vi "TimeTag_LSW_edits_June16.vi"() -> ()   [LabVIEW 2015]
doc: "This sample project is built upon the standard state machine template and shows how you could create an application that acquires, analyzes, and presents data. It includes functionality for presenting configuration dialogs, preserving settings between executions, loading and saving data, as well as exporting graph images and text files.\n\nIt is most appropriate for data that is acquired instantly as it does not allow for screen updates mid acquisition nor does it allow for continuous streaming to disk."
uses:
  <vilib>/ptbypt/NI_PtbyPt.lvlib
panel:
  in  "Averaging":dbl
  in  "Runs":dbl=100.0
  in  "Pulse TTL 2":bool
  in  "Pulse TTL 1":bool
  in  "Toggle\nTTL 2":bool
  in  "Toggle\nTTL 1":bool
  out "Total Starts":dbl
  in  "Record data":bool
  out "Initial time":dbl
  out "Elapsed time (s)":dbl
  out "FPGA_Run Status":dbl
  out "USB_Open Status":dbl
  out "Channel 4 Total\nCounts":dbl
  out "Channel 3 Total\nCounts":dbl
  out "Channel 2 Total\nCounts":dbl
  out "Channel 1 Total\nCounts":dbl
  in  "File Name":string="C:\\FPGA\\test.txt"
  out "?":dbl
  out "?":dbl
  out "?":dbl
  out "?":dbl
  out "stats":i64[](array[numeric])
  in  "Stop":bool
  out "Channel 4 CPS":dbl(knob) scale=0.0..600.0
  out "Channel 3 CPS":dbl(knob) scale=0.0..600.0
  out "Channel 2 CPS":dbl(knob) scale=0.0..600.0
  out "Channel 1 CPS":dbl(knob) scale=0.0..600.0
  # "Starts"
  # "Channel 1"
  # "Channel 2"
  # "Channel 3"
  # "Channel 4"
  # "Coincidence Channels 1 & 2"
  # "Coincidence Channels 1 & 3"
  # "Coincidence Channels 1 & 4"
  # "Coincidence Channels 2 & 3"
  # "Coincidence Channels 2 & 4"
  # "Coincidence Channels 3 & 4"
  # "Coincidence Channels 1 & 2 & 3"
  # "Coincidence Channels 1 & 2 & 4"
  # "Coincidence Channels 1 & 3 & 4"
  # "Coincidence Channels 2 & 3 & 4"
  # "Coincidence Channels 1 & 2 & 3 & 4"
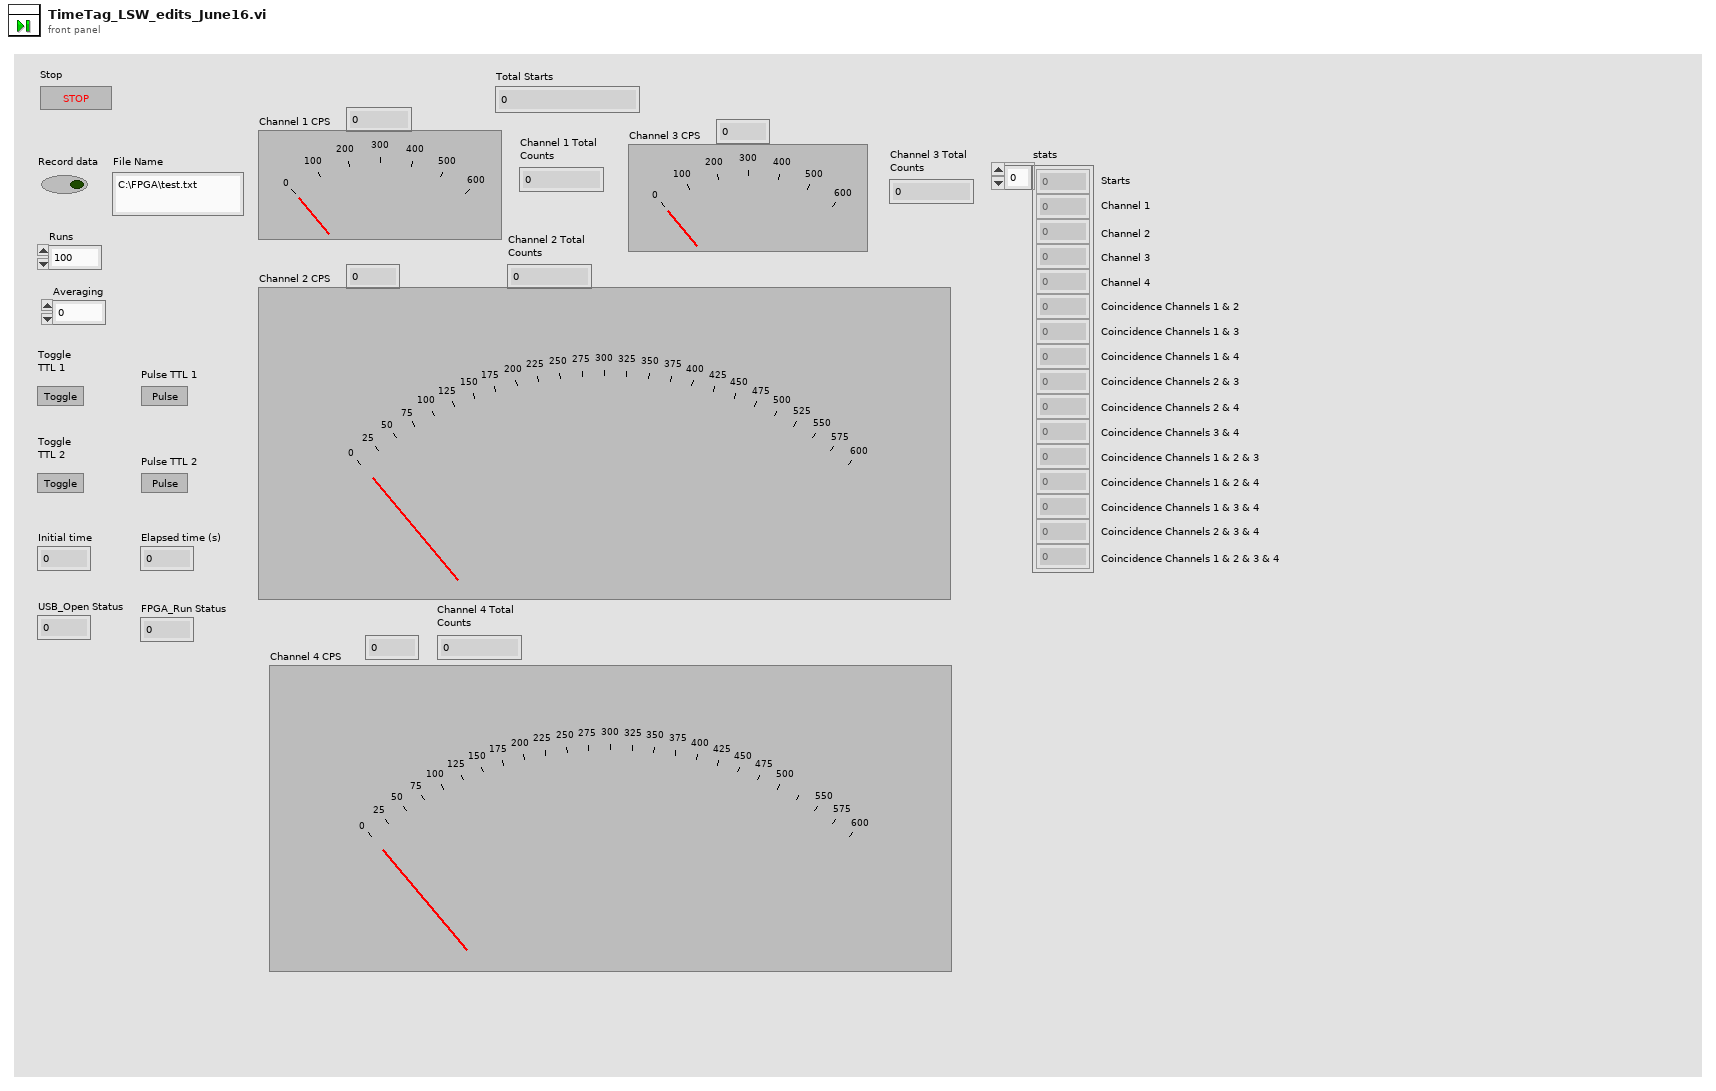
[diagram p1: front panel]
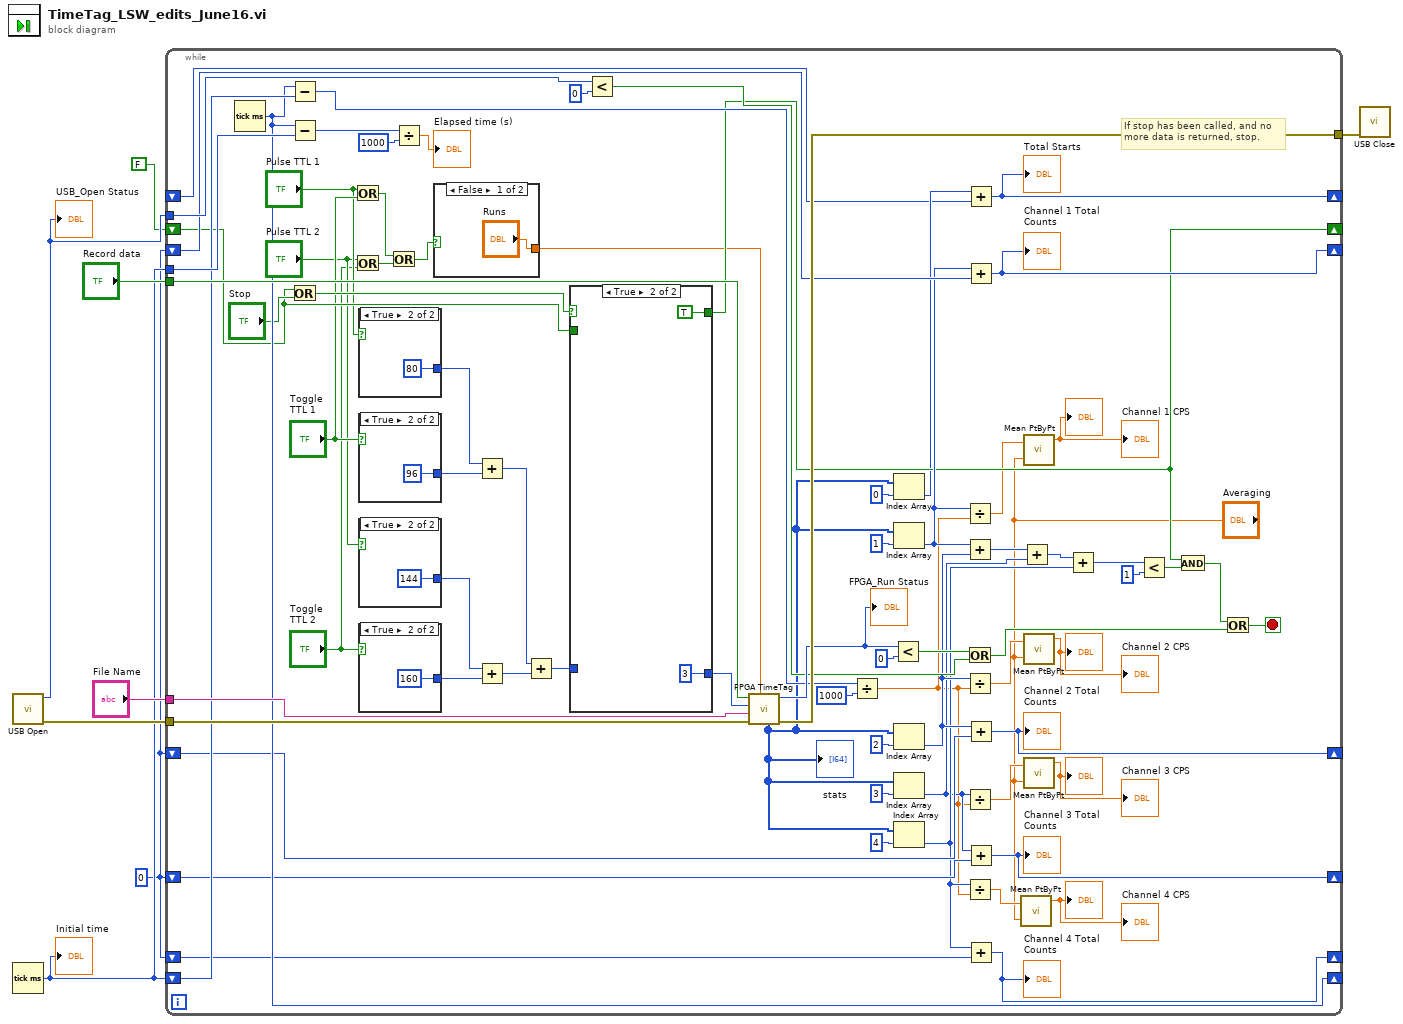
[diagram p0: block diagram]
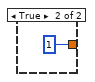
[diagram p2: hidden frame]
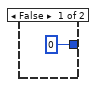
[diagram p3: hidden frame]
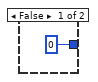
[diagram p4: hidden frame]
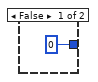
[diagram p5: hidden frame]
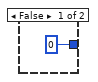
[diagram p6: hidden frame]
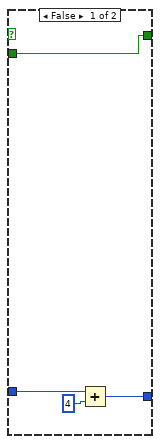
[diagram p7: hidden frame]
diagram:
  w2 = 0
  n1 = call "USB Open.vi"() -> ("error out"=w6:errorcluster, "function return"=w3:i32)  [unwired: 10 in]
  "USB_Open Status" <- w3
  n2 = Tick Count (ms)() -> (millisecond timer value=w4:u32)
  "Initial time" <- w4
  n3 = while {
    tunnel: w4 -> [w85]
    shift-right: [w62] -> _
    shift-left: w2 -> [w57]
    shift-right: [w61] -> _
    shift-left: w2 -> [w56]
    shift-right: [w60] -> _
    shift-left: w2 -> [w55]
    shift-right: [w53] -> _
    shift-left: w2 -> [w54]
    tunnel: w6 -> [w75]
    tunnel: [w76] -> w5
    tunnel: "Record data" -> [w73]
    tunnel: "File Name" -> [w74]
    shift-right: [w58] -> _
    shift-left: w4 -> [w70]
    tunnel: w3 -> [w66]
    shift-right: [w42] -> _
    shift-left: FALSE -> [w39]
    shift-right: [w33] -> _
    shift-left: _ -> [w35]
    stop <- w77 stop-if-true
    # "If stop has been called, and no\nmore data is returned, stop."
    n4 = Tick Count (ms)() -> (millisecond timer value=w58:u32)
    n5 = Subtract(x=w58, y=w70) -> (x-y=w69:u32)
    n6 = Subtract(x=w58, y=w85) -> (x-y=w84:u32)
    n7 = Or(x=w39, y="Stop") -> (x .or. y?=w41:bool)
    n8 = Or(x="Pulse TTL 1", y="Toggle\nTTL 1") -> (x .or. y?=w24:bool)
    n9 = Or(x="Pulse TTL 2", y="Toggle\nTTL 2") -> (x .or. y?=w25:bool)
    n10 = case shown="True" "Pulse TTL 1" {
      tunnel: [0 80] -> w32
      frame False {
      }
      frame True {
      }
    }
    n11 = case shown="True" "Toggle\nTTL 1" {
      tunnel: [0 96] -> w31
      frame False {
      }
      frame True {
      }
    }
    n12 = case shown="True" "Pulse TTL 2" {
      tunnel: [0 144] -> w28
      frame False {
      }
      frame True {
      }
    }
    n13 = case shown="True" "Toggle\nTTL 2" {
      tunnel: [0 160] -> w29
      frame False {
      }
      frame True {
      }
    }
    n14 = Or(x=w24, y=w25) -> (x .or. y?=w26:bool)
    n15 = Divide(x=w84, y=1000) -> (x/y=→"Elapsed time (s)":dbl)
    n16 = case shown="False" w26 {
      tunnel: ["Runs" 1] -> w22
      frame False {
      }
      frame True {
      }
    }
    n17 = Add(x=w32, y=w31) -> (x+y=w30:i32)
    n18 = Add(x=w28, y=w29) -> (x+y=w27:i32)
    n19 = Add(x=w30, y=w27) -> (x+y=w23:i32)
    n20 = case shown="True" w41 {
      tunnel: [w97 3] -> w59
      tunnel: [w99 TRUE] -> w42
      tunnel: w39 -> [w99 _]
      tunnel: w23 -> [w96 _]
      frame False {
        n21 = Add(x=w96, y=4) -> (x+y=w97:i32)
      }
      frame True {
      }
    }
    n22 = Less?(x=w66, y=0) -> (x < y?=w64:bool)
    n23 = call "FPGA TimeTag.vi"("runs"=w22, "error in (no error)"=w75, "fileName"=w74, "fpgaCommand"=w59, "saveData"=w73) -> ("error out"=w76:errorcluster, "function return"=w72:i32, "stats"=w36:i64[])  [unwired: 4 in]
    "stats" <- w36
    "FPGA_Run Status" <- w72
    n24 = Divide(x=w69, y=1000) -> (x/y=w34:dbl)
    n25 = Less?(x=w72, y=0) -> (x < y?=w65:bool)
    n26 = Index Array(array=w36, index=0) -> (element=w37:i64)
    n27 = Index Array(array=w36, index=1) -> (element=w45:i64)
    n28 = Index Array(array=w36, index=2) -> (element=w52:i64)
    n29 = Index Array(array=w36, index=3) -> (element=w48:i64)
    n30 = Index Array(array=w36, index=4) -> (element=w49:i64)
    n31 = Divide(x=w45, y=w34) -> (x/y=w17:dbl)
    n32 = Add(x=w45, y=w52) -> (x+y=w47:i64)
    n33 = Or(x=w65, y=w64) -> (x .or. y?=w63:bool)
    n34 = Divide(x=w52, y=w34) -> (x/y=w15:dbl)
    n35 = Divide(x=w48, y=w34) -> (x/y=w13:dbl)
    n36 = Divide(x=w49, y=w34) -> (x/y=w11:dbl)
    n37 = Add(x=w37, y=w35) -> (x+y=w33:i64)
    "Total Starts" <- w33
    n38 = Add(x=w45, y=w57) -> (x+y=w62:i64)
    "Channel 1 Total\nCounts" <- w62
    n39 = Add(x=w52, y=w56) -> (x+y=w61:i64)
    "Channel 2 Total\nCounts" <- w61
    n40 = Add(x=w48, y=w55) -> (x+y=w60:i64)
    "Channel 3 Total\nCounts" <- w60
    n41 = Add(x=w49, y=w54) -> (x+y=w53:i64)
    "Channel 4 Total\nCounts" <- w53
    n42 = call <vilib>:"Mean PtByPt.vi"("x"=w11, "sample length"="Averaging") -> ("mean"=→"Channel 4 CPS" →"?":dbl)  [unwired: 2 in, 1 out]
    n43 = Add(x=w47, y=w48) -> (x+y=w51:i64)
    n44 = call <vilib>:"Mean PtByPt.vi"("x"=w17, "sample length"="Averaging") -> ("mean"=→"Channel 1 CPS" →"?":dbl)  [unwired: 2 in, 1 out]
    n45 = call <vilib>:"Mean PtByPt.vi"("x"=w15, "sample length"="Averaging") -> ("mean"=→"Channel 2 CPS" →"?":dbl)  [unwired: 2 in, 1 out]
    n46 = call <vilib>:"Mean PtByPt.vi"("x"=w13, "sample length"="Averaging") -> ("mean"=→"Channel 3 CPS" →"?":dbl)  [unwired: 2 in, 1 out]
    n47 = Add(x=w51, y=w49) -> (x+y=w50:i64)
    n48 = Less?(x=w50, y=1) -> (x < y?=w44:bool)
    n49 = And(x=w42, y=w44) -> (x .and. y?=w43:bool)
    n50 = Or(x=w43, y=w63) -> (x .or. y?=w77:bool)
  }
  n51 = call "USB Close.vi"("error in (no error)"=w5) -> ()  [unwired: 9 in, 2 out]
